vi "generate table.vi"(7 "table":refnum<vi>, 8 "error in":errorcluster, 10 "engine configuration in":refnum<class "engine configuration.lvclass">, 11 "Scan Engine configuration":refnum<class "Scan Engine configuration.lvclass">) -> (0 "error out":errorcluster)   [LabVIEW 2013, in "Scan Engine editor node.lvclass"]
uses:
  Scan Engine editor node.lvclass
  <vilib>/NI/Module Execution Interface/Engine Configuration/engine configuration.lvclass
  module/configuration/Scan Engine configuration.lvclass
  <vilib>/NI/Configuration Framework/serializable configuration/NISE_CEF_serializable configuration.lvclass/NISE_CEF_serializable configuration.ctl
  <vilib>/NI/Configuration Framework/serializable configuration/NISE_CEF_serializable configuration.lvclass
  table line.ctl
  <vilib>/NI/Tag Bus Module Framework/channel/TBM channel.lvclass
  <vilib>/NI/Tag Bus/tag/tag descriptor.lvclass/tag descriptor.ctl
  <vilib>/NI/Tag Bus/tag/read tag name.vi
  <vilib>/NI/Configuration Framework/serializable configuration/Read UID.vi
  <vilib>/NI/Tag Bus/tag/tag descriptor.lvclass
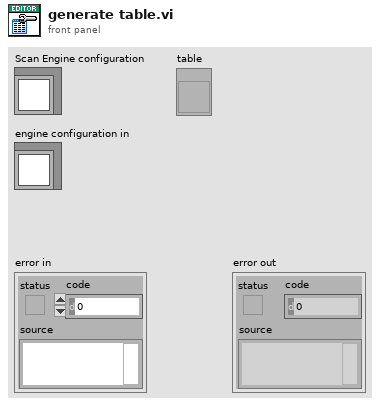
[diagram p1: front panel]
types:
  T1 = typedef "Scan Engine editor node.lvclass/table line.ctl" = cluster{"tag":string, "channel":refnum<class "TBM channel.lvclass">}
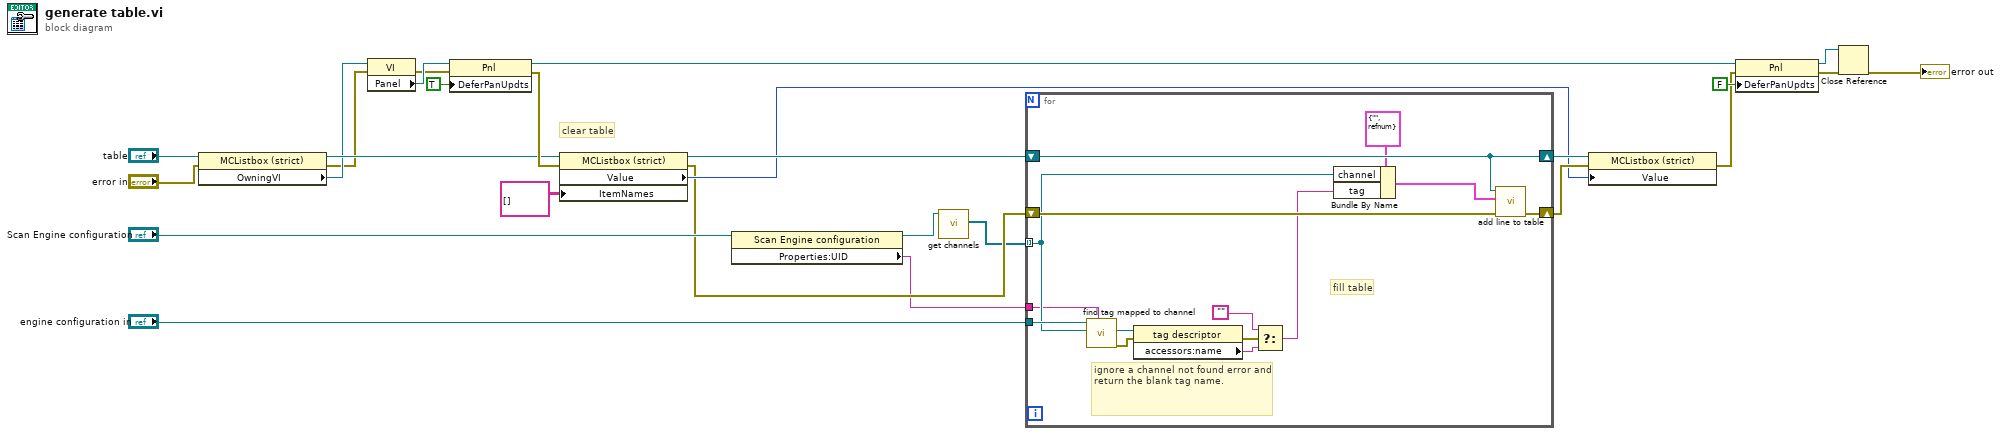
[diagram p0: block diagram]
diagram:
  # "clear table"
  n1 = property class="MCListbox (strict)"(reference="table", error in="error in") -> (reference out=w11:refnum<vi>, error out=w8:errorcluster, "OwningVI"=w9:refnum<vi>)
  n2 = property class="VI"(reference=w9, error in=w8) -> (error out=w17:errorcluster, "Panel"=w18:refnum<vi>)  [unwired: 1 out]
  n3 = property class="Pnl"(reference=w18, error in=w17, "DeferPanUpdts"=TRUE ("Defer Panel Updates")) -> (reference out=w14:refnum<vi>, error out=w16:errorcluster)
  n4 = property class="MCListbox (strict)"(reference=w11, error in=w16, "ItemNames"=string[][] [] ("Item Names")) -> (reference out=w25:refnum<vi>, error out=w4:errorcluster, "Value"=w20:i32)
  n5 = property class="Scan Engine configuration"(reference="Scan Engine configuration") -> (reference out=w2:refnum<class "Scan Engine configuration.lvclass">, "Properties:UID"=w3:string)  [unwired: 1 in, 1 out]
  n6 = call-dynamic "get channels.vi"("module configuration in"=w2) -> ("channels"=w1:refnum<class "TBM channel.lvclass">[])  [unwired: 9 in, 1 out]
  n7 = for {
    shift-right: [w40] -> w21
    shift-left: w4 -> [w39]
    tunnel: w1 -> [w33] mode=indexing
    tunnel: "engine configuration in" -> [w38]
    shift-right: [w36] -> w22
    shift-left: w25 -> [w36]
    tunnel: w3 -> [w32]
    # "ignore a channel not found error and return the blank tag name."
    # "fill table"
    n8 = call <vilib>:"find tag mapped to channel.vi"("owner"=w32, "channel"=w33, "engine configuration in"=w38) -> ("error out"=w31:errorcluster, "tag"=w37:refnum<class "tag descriptor.lvclass">)  [unwired: 6 in, 1 out]
    n9 = property class="tag descriptor"(reference=w37, error in=w31) -> (error out=w30:errorcluster, "accessors:name"=w29:string)  [unwired: 1 out]
    n10 = Select(t="", s=w30, f=w29) -> (s? t:f=w28:string)
    n11 = Bundle By Name(cluster=T1 {"tag"="", "channel"=refnum} ("line"), "channel"=w33, "tag"=w28) -> (w34:T1)
    n12 = call "add line to table.vi"("error in"=w39, "line"=w34, "operations table"=w36) -> ("error out"=w40:errorcluster)  [unwired: 8 in]
  }
  n13 = property class="MCListbox (strict)"(reference=w22, error in=w21, "Value"=w20) -> (error out=w13:errorcluster)  [unwired: 1 out]
  n14 = property class="Pnl"(reference=w14, error in=w13, "DeferPanUpdts"=FALSE ("Defer Panel Updates")) -> (reference out=w6:refnum<vi>, error out=w12:errorcluster)
  n15 = Close Reference(reference=w6, error in (no error)=w12) -> (error out=→"error out":errorcluster)
